vi "GetType&ID.vi"(8 "Error In":errorcluster, 10 "Plugin reference out":refnum<class "ModuleAdmin.lvclass">, 11 "PacificPowerSource in":refnum<class "PacificPowerSource.lvclass">) -> (0 "Error Out":errorcluster, 1 "Cluster":T1, 2 "reference out":refnum<class "ModuleAdmin.lvclass">, 3 "PacificPowerSource out":refnum<class "PacificPowerSource.lvclass">)   [LabVIEW 2018, in "AcPwrPlugins.lvlib" / "PacificPowerSource.lvclass"]
uses:
  PacificPowerSource.lvclass
  AcPwrBaseClass/AcPwrBase.lvclass
  <userlib>/NIST/ModuleAdminLib/ModuleAdmin/ModuleAdmin.lvclass
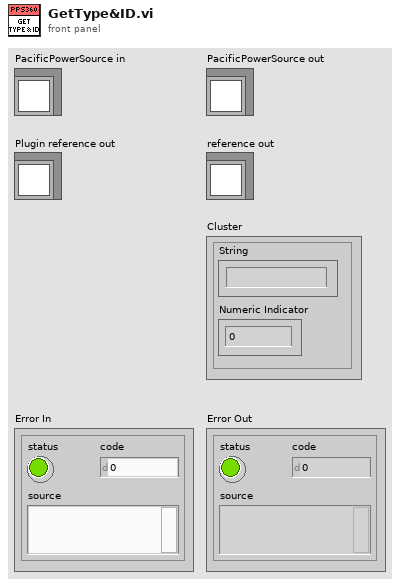
[diagram p1: front panel]
types:
  T1 = cluster{"String":string, "Numeric Indicator":i32}
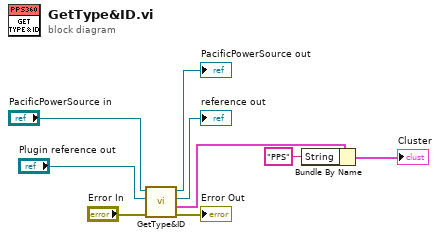
[diagram p0: block diagram]
diagram:
  n1 = call-parent "GetType&ID.vi"("Error In"="Error In", "Plugin reference out"="Plugin reference out", "AcPwrBase in"="PacificPowerSource in") -> ("Error Out"=→"Error Out":errorcluster, "Cluster"=w1:T1, "reference out"=→"reference out":refnum<class "ModuleAdmin.lvclass">, "AcPwrBase out"=→"PacificPowerSource out":refnum<class "PacificPowerSource.lvclass">)  [unwired: 5 in]
  n2 = Bundle By Name(cluster=w1, "String"="PPS") -> (→"Cluster":T1)
